vi "rs3_ExtractColor3.vi"(0 "Depth X":i32=480, 1 "Depth Y":i32=360, 2 "X offset":dbl, 4 "RGB Y":i32=480, 5 "Alpha":dbl, 6 "RGB  X":i32=640, 7 "24bit Color Array":u8[](array[numeric]), 8 "Blue":dbl=2.0, 9 "Green":dbl=1.0, 10 "Red":dbl=2.0, 11 "White Balance":bool) -> (3 "Norm Mesh Color":T1(array[cluster]))   [LabVIEW 2017, in "libRealSense3.lvlib"]
doc: "Extract the color in a format required for plotting a pointcloud into 3D picture indication"
uses:
  <vilib>/addons/RealSense/libRealSense3.lvlib
panel:
  out "Ratio X":dbl=1.3333333333333333
  out "Ratio Y":dbl=1.3333333333333333
  # "RS3 Extract Color for PointCloud"
  # "(C) Intel Corp. 2017,  AGJ"
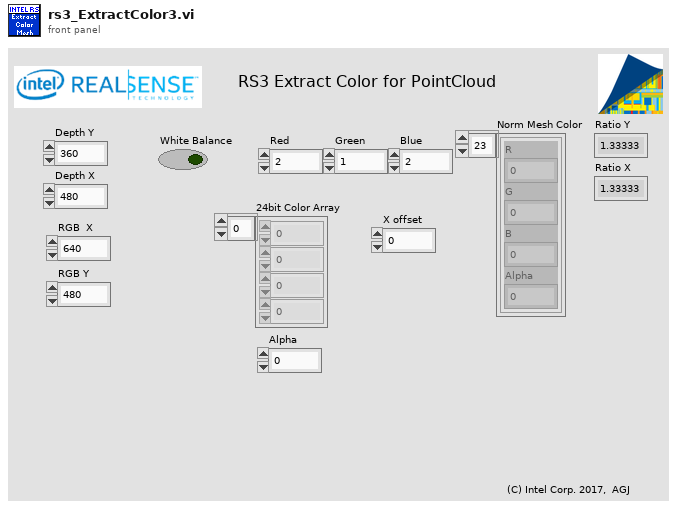
[diagram p1: front panel]
types:
  T1 = cluster{"R":dbl, "G":dbl, "B":dbl, "Alpha":dbl}[]
  T2 = cluster{"upper limit":dbl, "upper limit":dbl, "upper limit":dbl, "Alpha":dbl}[]
  T3 = cluster{"upper limit":dbl, "upper limit":dbl, "upper limit":dbl, "Alpha":dbl}
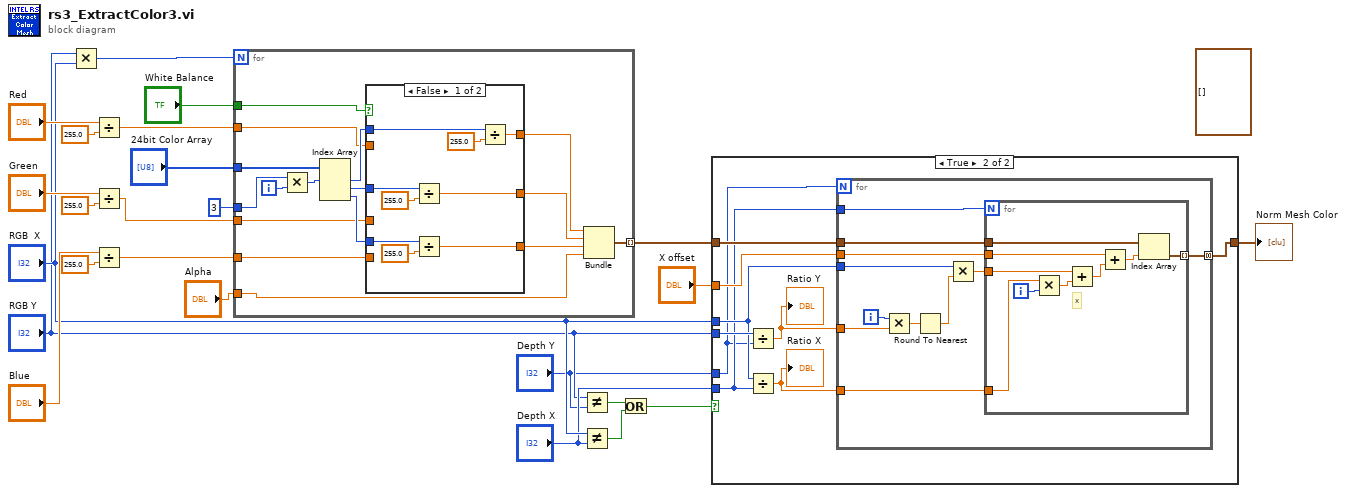
[diagram p0: block diagram]
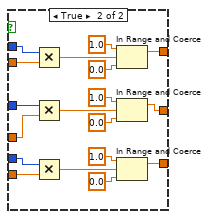
[diagram p3: hidden frame]
diagram:
  (unwired) T2 []
  n1 = Multiply(x="RGB Y", y="RGB  X") -> (x*y=w12:i32)
  n2 = Divide(x="Red", y=255.0 ("upper limit")) -> (x/y=w20:dbl)
  n3 = Divide(x="Green", y=255.0 ("upper limit")) -> (x/y=w14:dbl)
  n4 = Divide(x="Blue", y=255.0 ("upper limit")) -> (x/y=w15:dbl)
  n5 = for {
    N: w12 -> [_]
    tunnel: "24bit Color Array" -> [w38]
    tunnel: 3 ("# of bytes/number") -> [w37]
    tunnel: [w36] -> w11 mode=indexing
    tunnel: w20 -> [w32]
    tunnel: w14 -> [w31]
    tunnel: w15 -> [w30]
    tunnel: "Alpha" -> [w26]
    tunnel: "White Balance" -> [w25]
    i -> [w40]
    n6 = Multiply(x=w37, y=w40) -> (x*y=w39:i32)
    n7 = Index Array(array=w38, index #1=w39) -> (element #1=w35:u8, element #2=w34:u8, element #3=w33:u8)  [unwired: 2 in]
    n8 = case shown="False" w25 {
      tunnel: w35 -> [w48 w67]
      tunnel: w34 -> [w44 w66]
      tunnel: w33 -> [w43 w65]
      tunnel: w32 -> [_ w64]
      tunnel: w31 -> [_ w63]
      tunnel: w30 -> [_ w62]
      tunnel: [w47 w52] -> w29
      tunnel: [w41 w51] -> w28
      tunnel: [w42 w50] -> w27
      frame False {
        n9 = Divide(x=w44, y=255.0 ("upper limit")) -> (x/y=w41:dbl)
        n10 = Divide(x=w43, y=255.0 ("upper limit")) -> (x/y=w42:dbl)
        n11 = Divide(x=w48, y=255.0 ("upper limit")) -> (x/y=w47:dbl)
      }
      frame True {
        n12 = Multiply(x=w67, y=w64) -> (x*y=w61:dbl)
        n13 = Multiply(x=w66, y=w63) -> (x*y=w55:dbl)
        n14 = Multiply(x=w65, y=w62) -> (x*y=w56:dbl)
        n15 = In Range and Coerce(upper limit=1.0, x=w61, lower limit=0.0) -> (coerced(x)=w52:dbl)  [unwired: 1 out]
        n16 = In Range and Coerce(upper limit=1.0, x=w55, lower limit=0.0) -> (coerced(x)=w51:dbl)  [unwired: 1 out]
        n17 = In Range and Coerce(upper limit=1.0, x=w56, lower limit=0.0) -> (coerced(x)=w50:dbl)  [unwired: 1 out]
      }
    }
    n18 = Bundle("upper limit"=w29, "upper limit"=w28, "upper limit"=w27, "Alpha"=w26) -> (w36:T3)  [unwired: 1 in]
  }
  n19 = Not Equal?(x="RGB Y", y="Depth Y") -> (x != y?=w4:bool)
  n20 = Not Equal?(x="RGB  X", y="Depth X") -> (x != y?=w7:bool)
  n21 = Or(x=w4, y=w7) -> (x .or. y?=w3:bool)
  n22 = case shown="True" w3 {
    tunnel: w11 -> [w68 w77]
    tunnel: [w68 w76] -> w1
    tunnel: "RGB Y" -> [_ w75]
    tunnel: "X offset" -> [_ w74]
    tunnel: "RGB  X" -> [_ w73]
    tunnel: "Depth X" -> [_ w72]
    tunnel: "Depth Y" -> [_ w71]
    frame False {
    }
    frame True {
      n23 = Divide(x=w75, y=w71) -> (x/y=w69:dbl)
      "Ratio Y" <- w69
      n24 = Divide(x=w73, y=w72) -> (x/y=w70:dbl)
      "Ratio X" <- w70
      n25 = for {
        N: w71 -> [_]
        tunnel: w72 -> [w88]
        tunnel: w70 -> [w87]
        tunnel: w69 -> [w84]
        tunnel: w73 -> [w80]
        tunnel: w77 -> [w86]
        tunnel: [w85] -> w76 mode=concatenating
        tunnel: w74 -> [w78]
        i -> [w82]
        n26 = Multiply(x=w82, y=w84) -> (x*y=w83:dbl)
        n27 = Round To Nearest(number=w83) -> (nearest integer value=w81:dbl)
        n28 = Multiply(x=w80, y=w81) -> (x*y=w79:dbl)
        n29 = for {
          N: w88 -> [_]
          tunnel: w87 -> [w96]
          tunnel: w86 -> [w94]
          tunnel: [w93] -> w85 mode=indexing
          tunnel: w79 -> [w92]
          tunnel: w78 -> [w90]
          i -> [w97]
          # "x"
          n30 = Multiply(x=w96, y=w97) -> (x*y=w95:dbl)
          n31 = Add(x=w92, y=w95) -> (x+y=w91:dbl)
          n32 = Add(x=w90, y=w91) -> (x+y=w89:dbl)
          n33 = Index Array(array=w94, index=w89) -> (element=w93:T3)
        }
      }
    }
  }
  "Norm Mesh Color" <- w1
